vi "Test-P-R.vi"() -> ()   [LabVIEW 2013]
panel:
  out "Graph":cluster{dbl[unit], dbl[unit]}[](graph)
  in  "Stop Button":bool
  out "Chart":cluster{dbl, dbl}(graph)
  out "R":dbl[unit]
  out "P":dbl[unit]
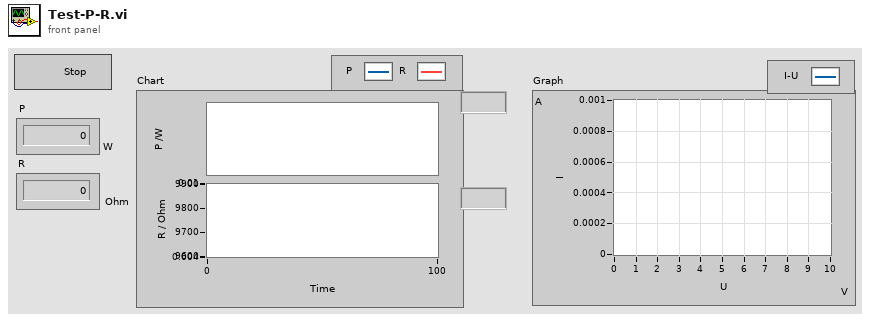
[diagram p1: front panel]
types:
  T1 = cluster{"Read Access":enum8{"Allowed", "Required", "None"}, "Write Access":enum8{"Allowed", "Required", "None"}}
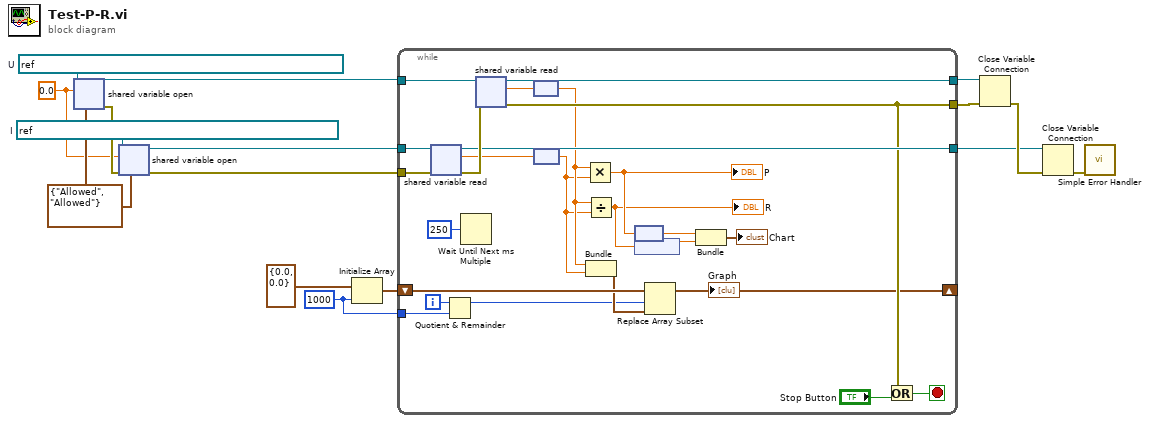
[diagram p0: block diagram]
diagram:
  w1 = 1000 ("dimension size")
  w12 = 0.0
  w13 = T1 {"Read Access"=enum."Allowed", "Write Access"=enum."Allowed"} ("access")
  w15 = refnum<k21> "ni.var.psp://localhost/SVTest/myDMM-KE2700_Reading"  # I
  w16 = refnum<k21> "ni.var.psp://localhost/SVTest/myDMM-Fluke45_Reading"  # U
  n1 = shared-variable-open(w16, w12, w13) -> (w9:refnum<k21>, w14:errorcluster)  [unwired: 1 in]
  n2 = shared-variable-open(w15, w14, w12, w13) -> (w11:refnum<k21>, w10:errorcluster)
  n3 = Initialize Array(cluster{dbl[unit], dbl[unit]} {0.0, 0.0} ("output cluster"), w1) -> (w2:cluster{dbl[unit], dbl[unit]}[])
  n4 = while {
    tunnel: w11 -> [w41]
    tunnel: w10 -> [w40]
    tunnel: w9 -> [w38]
    tunnel: [w30] -> w8
    tunnel: [w37] -> w6
    tunnel: [w36] -> w5
    shift-right: [w17] -> _
    shift-left: w2 -> [w22]
    tunnel: w1 -> [w19]
    i -> [w20]
    stop <- w31 stop-if-true
    n5 = shared-variable-read(w41, w40) -> (w36:refnum<k21>, w39:errorcluster, w27:dbl)  [unwired: 1 out]
    n6 = Quotient & Remainder(x=w20, y=w19) -> (x-y*floor(x/y)=w18:i32)  [unwired: 1 out]
    n7 = Wait Until Next ms Multiple(millisecond multiple=u32 250) -> ()  [unwired: 1 out]
    n8 = shared-variable-read(w38, w39) -> (w37:refnum<k21>, w30:errorcluster, w34:dbl)  [unwired: 1 out]
    n9 = node(w34) -> (w24:dbl[unit])
    n10 = node(w27) -> (w23:dbl[unit])
    n11 = Multiply(x=w24, y=w23) -> (x*y=w28:dbl[unit])
    "P" <- w28
    n12 = Divide(x=w24, y=w23) -> (x/y=w25:dbl[unit])
    "R" <- w25
    n13 = Bundle(w24, w23) -> (w21:cluster{dbl[unit], dbl[unit]})  [unwired: 1 in]
    n14 = node(w28) -> (w29:dbl)
    n15 = node(w25) -> (w26:dbl)
    n16 = Replace Array Subset(array=w22, new element=w21, index=w18) -> (w17:cluster{dbl[unit], dbl[unit]}[])
    "Graph" <- w17
    n17 = Bundle(w29, w26) -> (→"Chart":cluster{dbl, dbl})  [unwired: 1 in]
    n18 = Or(x=w30, y="Stop Button") -> (x .or. y?=w31:bool)
  }
  n19 = Close Variable Connection(8:w8, 11:w6) -> (0:w7:errorcluster)
  n20 = Close Variable Connection(8:w7, 11:w5) -> (0:w4:errorcluster)
  n21 = call <vilib>:"Simple Error Handler.vi"("error in (no error)"=w4) -> ()  [unwired: 4 in, 5 out]
